vi "Profile Coordinate Controls.vi"() -> ()   [LabVIEW 2015]
panel:
  in  "LongProf.Coords":T1(array[cluster])=[{"X0"=-72.9, "Y"=-56.5, "Z"=0.0, "Name"="Anemo1", "Spacing"=enum."Specified", "X.start"=45.0, "X.end"=45.0, "NumPts"=0.0}, {"X0"=-458.4, "Y"=87.9, "Z"=12.9, "Name"="Anemo2", "Spacing"=enum."Specified", "X.start"=45.0, "X.end"=45.0, "NumPts"=0.0}]
  in  "LatProf.Coords":T2(array[cluster])=[{"X"=-72.9, "Y0"=-56.5, "Z"=0.0, "Name"="Anemo1", "Spacing"=enum."Specified", "Y.start"=45.0, "Y.end"=45.0, "NumPts"=0.0}, {"X"=-458.4, "Y0"=87.9, "Z"=12.9, "Name"="Anemo2", "Spacing"=enum."Specified", "Y.start"=45.0, "Y.end"=45.0, "NumPts"=0.0}]
  in  "VertProf.Coords":T3(array[cluster])=[{"X"=-72.9, "Y"=-56.5, "Z0"=0.0, "Name"="Anemo1", "Spacing"=enum."Specified", "Z.start"=45.0, "Z.end"=45.0, "NumPts"=0.0}, {"X"=-458.4, "Y"=87.9, "Z0"=12.9, "Name"="Anemo2", "Spacing"=enum."Specified", "Z.start"=45.0, "Z.end"=45.0, "NumPts"=0.0}]
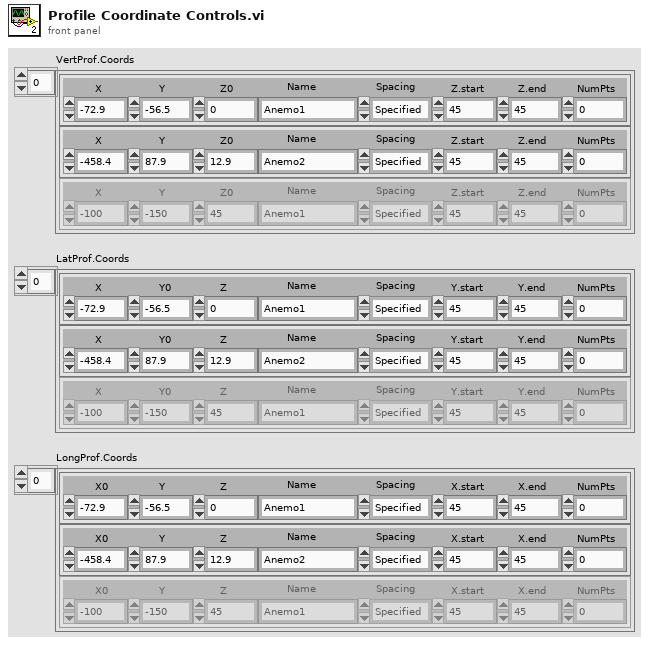
[diagram p1: front panel]
types:
  T1 = cluster{"X0":dbl, "Y":dbl, "Z":dbl, "Name":string, "Spacing":enum16{"Linear", "Log", "Gauss", "Specified", "N/A"}, "X.start":dbl, "X.end":dbl, "NumPts":dbl}[]
  T2 = cluster{"X":dbl, "Y0":dbl, "Z":dbl, "Name":string, "Spacing":enum16{"Linear", "Log", "Gauss", "Specified", "N/A"}, "Y.start":dbl, "Y.end":dbl, "NumPts":dbl}[]
  T3 = cluster{"X":dbl, "Y":dbl, "Z0":dbl, "Name":string, "Spacing":enum16{"Linear", "Log", "Gauss", "Specified", "N/A"}, "Z.start":dbl, "Z.end":dbl, "NumPts":dbl}[]
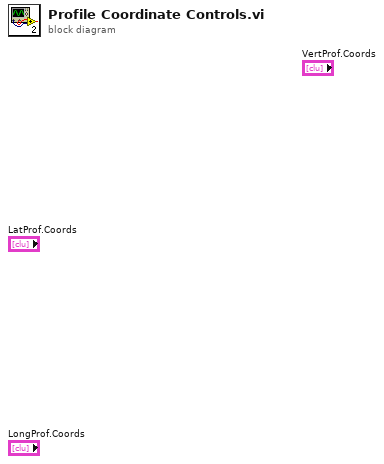
[diagram p0: block diagram]
diagram:
